vi "Set Position Setpoint.vi"(8 "error in (no error)":errorcluster, 10 "CCW position (rad)":dbl, 11 "KUKA youBot arm motor in":refnum<class "NI_Robotics_KUKA youBot Arm Motor.lvclass">) -> (0 "error out":errorcluster, 3 "KUKA youBot arm motor out":refnum<class "NI_Robotics_KUKA youBot Arm Motor.lvclass">)   [LabVIEW 2017, in "NI_Robotics_KUKA youBot Host.lvlib" / "NI_Robotics_KUKA youBot Arm Motor.lvclass"]
uses:
  <vilib>/robotics/KUKA youBot/Motor/Arm Motor/NI_Robotics_KUKA youBot Arm Motor.lvclass
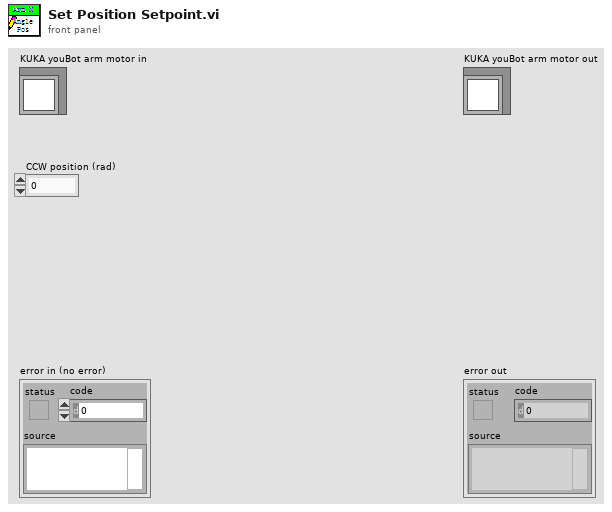
[diagram p1: front panel]
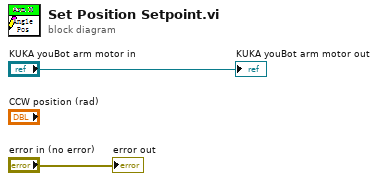
[diagram p0: block diagram]
diagram:
  "error out" <- "error in (no error)"
  "KUKA youBot arm motor out" <- "KUKA youBot arm motor in"
